vi "Curtin1_ViewType.vi"(10 "Settings":T2 {"mag/phase" items=["FRF", "rad phase unwrapped", "deg phase unwrapped", "rad phase wrapped", "deg phase wrapped", "White Plots", "MJ Map", "Real and Imaginary"]; "Bands" items=["No Bands", "", "Test2", "test3", "Test"]; "Smoothing" items=["No smoothing"=0, "1/4 semitone"=25, "1/2 semitone"=50, "1 semitone"=100, "2 semitones"=200, "Woodhouse"=19]; "View Type" items=["As measured", "Normalize", "Separate", "Complex Average", "Real Average", "Standard Deviation"]}, 11 "FRF in":cluster{dbl, "df":dbl, cdb[]}[](array[cluster])) -> (0 "Complex Out":cluster{dbl, "df":dbl, cdb[]}[](array[cluster]), 3 "FRF Out":cluster{"x0":dbl, "df":dbl, dbl[]}[](graph))   [LabVIEW 2022 SP3]
uses:
  GraphType.ctl
  Mic/Mic_Global.vi
  <vilib>/Analysis/NI_AALBase.lvlib
panel:
  out "Waveform Graph":cluster{dbl, "df":dbl, dbl[]}[](graph)
  out "Array":dbl[](array[numeric])
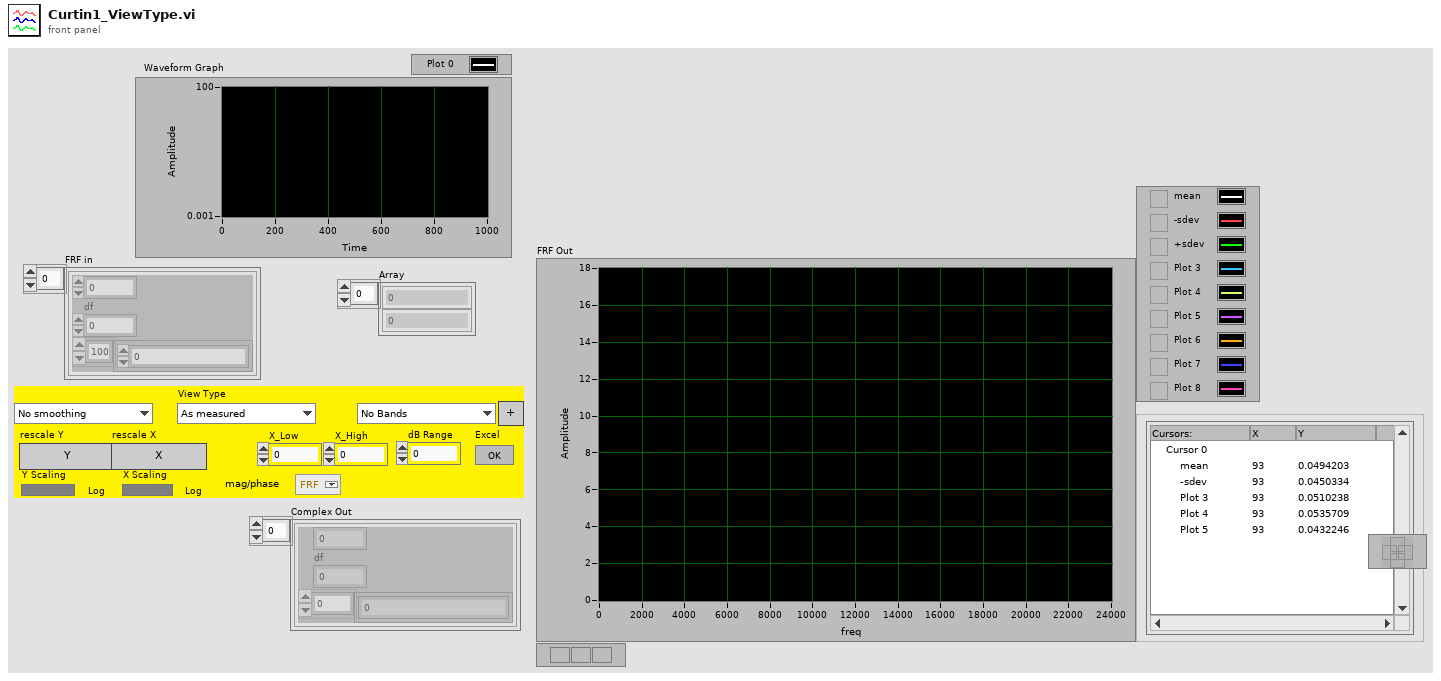
[diagram p1: front panel]
types:
  T1 = typedef "GraphType.ctl" = u16
  T2 = cluster{"View Type":u16, "Smoothing":u16, "Bands":u16, "New Band":bool, "rescale Y":bool, "rescale X":bool, "X_Low":dbl, "X_High":dbl, "dB Range":dbl, "Excel":bool, "Y Scaling":bool, "X Scaling":bool, "mag/phase":T1}
  T3 = cluster{"Alerts":bool, "Log X Axis":bool, "dB scale":bool, "Averaging":bool, "Fade":dbl, "Centroids?":bool, "line thickness":u8}
  T4 = typedef "PreferencesControl.ctl" = cluster{"Name of test":string, "Date":timestamp, "Location":string, "Template":string, "Soundcard":string, "resolution":u16, "Sampling rate":u16, "Ch1 Gain ":dbl, "Ch2 Gain":dbl, "Sample time (s)":dbl, "Pre-trigger (s)":dbl, "Hammer Threshold":dbl, "Positions":i16, "Taps/Position":i16, "Set Names":string, "Freq resolution":dbl, "Hammer cutoff":dbl, "Mic cutoff":dbl, "Double bounce ":dbl, "Hammer Cal":dbl, "dB Offset":dbl, "Accel Cal":dbl, "Vibrometer Cal":dbl, "Mic Cal":dbl, "Output":u16, "Voltage Cal":dbl, "Vibrometer Port":refnum<visa-resource-name>, "Range":u16, "High Pass":u16, "Bandwidth":u16, "X Range":cluster{"Minimum":dbl, "Maximum":dbl, "Increment":dbl, "Minor Increment":dbl, "Start":dbl}[], "Y Range":cluster{"Minimum":dbl, "Maximum":dbl, "Increment":dbl, "Minor Increment":dbl, "Start":dbl}[], "dB Spread":dbl, "Trigger":u16, "Ch_1":u8, "Ch_2":u8, "flip?":bool, "60Hz":bool, "Time offset":dbl, "Piezo Cal":dbl, "Default Notes":string}
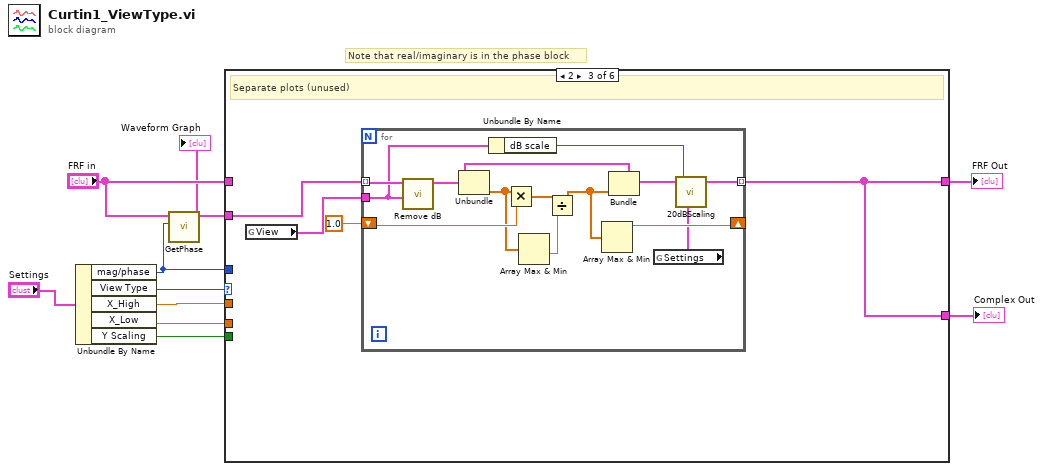
[diagram p0: block diagram]
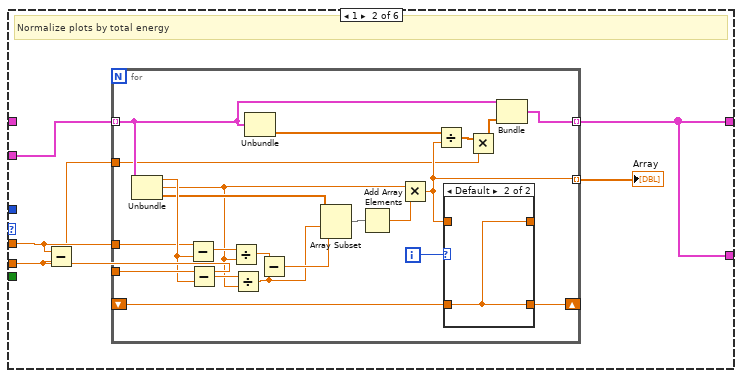
[diagram p3: hidden frame]
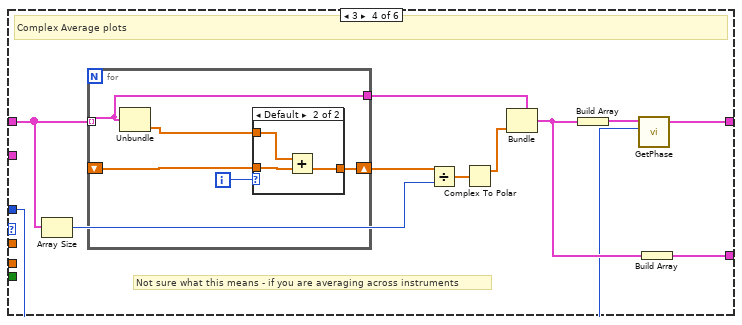
[diagram p5: hidden frame]
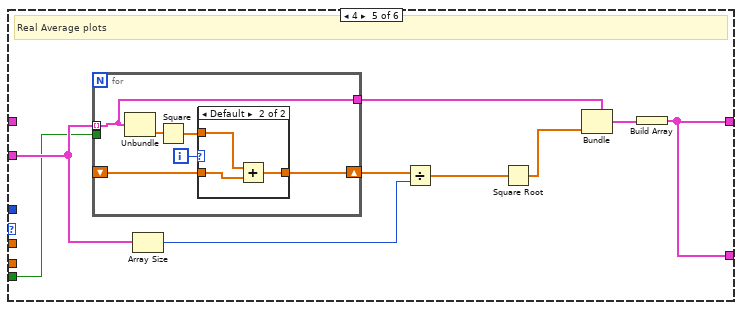
[diagram p7: hidden frame]
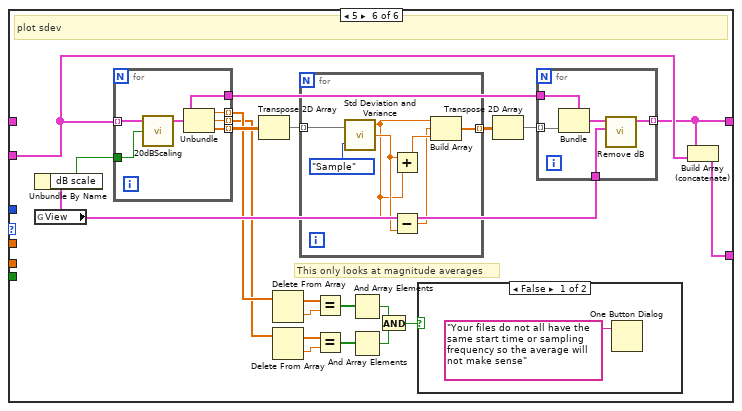
[diagram p9: hidden frame]
diagram:
  # "Note that real/imaginary is in the phase block"
  n1 = Unbundle By Name("Settings") -> ("mag/phase"=w4:T1, "View Type"=w9:u16, "X_High"=w7:dbl, "X_Low"=w8:dbl, "Y Scaling"=w3:bool)
  n2 = call "GetPhase.vi"("mag/phase"=w4, "FRF in"="FRF in") -> ("Array"=w1:cluster{dbl, "df":dbl, dbl[]}[])  [unwired: 9 in]
  "Waveform Graph" <- w1
  n3 = case shown="2" w9 {
    tunnel: "FRF in" -> [w12 _ _ w68 _ _]
    tunnel: [w11 w17 w44 w63 w82 w99] -> w2
    tunnel: w7 -> [_ w16 _ _ _ _]
    tunnel: w8 -> [_ w15 _ _ _ _]
    tunnel: [w12 w17 w44 w66 w82 w100] -> w6
    tunnel: w1 -> [w11 w13 w43 _ w81 w101]
    tunnel: w4 -> [_ _ _ w62 _ _]
    tunnel: w3 -> [_ _ _ _ w80 _]
    frame 0, Default {
    }
    frame 1 {
      # "Normalize plots by total energy"
      n4 = Subtract(x=w16, y=w15) -> (x-y=w14:dbl)
      n5 = for {
        tunnel: w13 -> [w20] mode=indexing
        tunnel: [w40] -> w17 mode=indexing
        tunnel: w15 -> [w28]
        tunnel: w16 -> [w27]
        shift-right: [w25] -> _
        shift-left: _ -> [w24]
        tunnel: [w21] -> w18 mode=indexing
        tunnel: w14 -> [w19]
        i -> [w26]
        n6 = Unbundle(w20) -> (w35:dbl, "df"=w23:dbl, w30:dbl[])
        n7 = Subtract(x=w27, y=w35) -> (x-y=w34:dbl)
        n8 = Subtract(x=w28, y=w35) -> (x-y=w36:dbl)
        n9 = Divide(x=w34, y=w23) -> (x/y=w29:dbl)
        n10 = Divide(x=w36, y=w23) -> (x/y=w31:dbl)
        n11 = Unbundle(w20) -> (w39:dbl[])  [unwired: 2 out]
        n12 = Subtract(x=w29, y=w31) -> (x-y=w32:dbl)
        n13 = Array Subset(array=w30, index=w31, length=w32) -> (w33:dbl[])
        n14 = Add Array Elements(numeric array=w33) -> (sum=w22:dbl)
        n15 = Multiply(x=w23, y=w22) -> (x*y=w21:dbl)
        n16 = Divide(x=w39, y=w21) -> (x/y=w38:dbl[])
        n17 = case shown="Default" w26 {
          tunnel: [w41 w42] -> _
          tunnel: w21 -> [w41 _]
          tunnel: [w41 w42] -> w25
          tunnel: w24 -> [_ w42]
          frame 0 {
          }
          frame Default {
          }
        }
        n18 = Multiply(x=w38, y=w19) -> (x*y=w37:dbl[])
        n19 = Bundle(cluster=w20, w37) -> (w40:cluster{dbl, "df":dbl, dbl[]})  [unwired: 2 in]
      }
      "Array" <- w18
    }
    frame 2 {
      # "Separate plots (unused)"
      n20 = global read "Mic_Global.vi" "View"() -> (w45:T3)
      n21 = for {
        tunnel: w43 -> [w56] mode=indexing
        shift-right: [w57] -> _
        shift-left: 1.0 -> [w59]
        tunnel: [w53] -> w44 mode=indexing
        tunnel: w45 -> [w52]
        n22 = call "Remove dB.vi"("View"=w52, "Average FRF in"=w56) -> ("Average FRF out"=w55:cluster{"x0":dbl, "df":dbl, dbl[]})  [unwired: 9 in]
        n23 = Unbundle(w55) -> (w49:dbl[])  [unwired: 2 out]
        n24 = Unbundle By Name(w52) -> ("dB scale"=w51:bool)
        n25 = Multiply(x=w49, y=w59) -> (x*y=w58:dbl[])
        n26 = Array Max & Min(array=w49) -> (min value=w50:dbl)  [unwired: 3 out]
        n27 = Divide(x=w58, y=w50) -> (x/y=w48:dbl[])
        n28 = Array Max & Min(array=w48) -> (max value=w57:dbl)  [unwired: 3 out]
        n29 = Bundle(cluster=w55, w48) -> (w54:cluster{"x0":dbl, "df":dbl, dbl[]})  [unwired: 2 in]
        n30 = global read "Mic_Global.vi" "Settings"() -> (w47:T4)
        n31 = call "20dBScaling.vi"("Average FRF in"=w54, "dB?"=w51, "Settings"=w47) -> ("Average FRF out"=w53:cluster{"x0":dbl, "df":dbl, dbl[]})  [unwired: 3 in, 1 out]
      }
    }
    frame 3 {
      # "Not sure what this means - if you are averaging across instruments"
      # "Complex Average plots"
      n32 = Array Size(array=w68) -> (size(s)=w67:i32)
      n33 = for {
        tunnel: w68 -> [w75] mode=indexing
        tunnel: [w75] -> w70
        shift-right: [w73] -> w69
        shift-left: _ -> [w72]
        i -> [w74]
        n34 = Unbundle(w75) -> (w71:cdb[])  [unwired: 2 out]
        n35 = case shown="Default" w74 {
          tunnel: [w76 w77] -> w73
          tunnel: w71 -> [w76 w78]
          tunnel: w72 -> [_ w79]
          frame 0 {
          }
          frame Default {
            n36 = Add(x=w78, y=w79) -> (x+y=w77:cdb[])
          }
        }
      }
      n37 = Divide(x=w69, y=w67) -> (x/y=w61:cdb[])
      n38 = Complex To Polar(r * e^(i*theta)=w61) -> (r=w60:dbl[])  [unwired: 1 out]
      n39 = Bundle(cluster=w70, w60) -> (w65:cluster{dbl, "df":dbl, cdb[]})  [unwired: 2 in]
      n40 = Build Array(w65) -> (w64:cluster{dbl, "df":dbl, cdb[]}[])
      n41 = call "GetPhase.vi"("mag/phase"=w62, "FRF in"=w64) -> ("Array"=w63:cluster{dbl, "df":dbl, dbl[]}[])  [unwired: 9 in]
      n42 = Build Array(w65) -> (w66:cluster{dbl, "df":dbl, cdb[]}[])
    }
    frame 4 {
      # "Real Average plots"
      n43 = for {
        tunnel: w81 -> [w89] mode=indexing
        tunnel: [w89] -> w88
        shift-right: [w93] -> w87
        shift-left: _ -> [w91]
        tunnel: w80 -> [_]
        i -> [w94]
        n44 = Unbundle(w89) -> (w92:dbl[])  [unwired: 2 out]
        n45 = Square(x=w92) -> (x^2=w90:dbl[])
        n46 = case shown="Default" w94 {
          tunnel: [w95 w96] -> w93
          tunnel: w90 -> [w95 w97]
          tunnel: w91 -> [_ w98]
          frame 0 {
          }
          frame Default {
            n47 = Add(x=w97, y=w98) -> (x+y=w96:dbl[])
          }
        }
      }
      n48 = Array Size(array=w81) -> (size(s)=w86:i32)
      n49 = Divide(x=w87, y=w86) -> (x/y=w85:dbl[])
      n50 = Square Root(x=w85) -> (sqrt(x)=w83:dbl[])
      n51 = Bundle(cluster=w88, w83) -> (w84:cluster{dbl, "df":dbl, dbl[]})  [unwired: 2 in]
      n52 = Build Array(w84) -> (w82:cluster{dbl, "df":dbl, dbl[]}[])
    }
    frame 5 {
      # "This only looks at magnitude averages"
      # "plot sdev"
      n53 = global read "Mic_Global.vi" "View"() -> (w115:T3)
      n54 = Unbundle By Name(w115) -> ("dB scale"=w116:bool)
      n55 = for {
        tunnel: w101 -> [w134] mode=indexing
        tunnel: [w133] -> w119
        tunnel: [w138] -> w118 mode=indexing
        tunnel: w116 -> [w137]
        tunnel: [w136] -> w112 mode=indexing
        tunnel: [w135] -> w105 mode=indexing
        n56 = call "20dBScaling.vi"("Average FRF in"=w134, "dB?"=w137) -> ("Average FRF out"=w133:cluster{"x0":dbl, "df":dbl, dbl[]})  [unwired: 4 in, 1 out]
        n57 = Unbundle(w133) -> ("x0"=w136:dbl, "df"=w135:dbl, w138:dbl[])
      }
      n58 = Transpose 2D Array(2D array=w118) -> (transposed array=w114:dbl[][])
      n59 = Delete From Array(array=w112) -> (deleted portion=w111:dbl, array with subset deleted=w110:dbl[])  [unwired: 2 in]
      n60 = Delete From Array(array=w105) -> (deleted portion=w106:dbl, array with subset deleted=w107:dbl[])  [unwired: 2 in]
      n61 = for {
        tunnel: w114 -> [w132] mode=indexing
        tunnel: [w128] -> w113 mode=indexing
        n62 = call <vilib>:"Std Deviation and Variance.vi"("X"=w132, "Weighting (Sample)"=enum16{"Sample", "Population"}."Sample") -> ("mean"=w129:dbl, "standard deviation"=w131:dbl)  [unwired: 1 out]
        n63 = Add(x=w131, y=w129) -> (x+y=w127:dbl)
        n64 = Subtract(x=w129, y=w131) -> (x-y=w126:dbl)
        n65 = Build Array(w129, w126, w127) -> (w128:dbl[])
      }
      n66 = Equal?(x=w110, y=w111) -> (x = y?=w109:bool[])
      n67 = Equal?(x=w107, y=w106) -> (x = y?=w108:bool[])
      n68 = And Array Elements(Boolean array=w109) -> (logical AND=w104:bool)
      n69 = And Array Elements(Boolean array=w108) -> (logical AND=w103:bool)
      n70 = And(x=w104, y=w103) -> (x .and. y?=w102:bool)
      n71 = case shown="False" w102 {
        frame False {
          n72 = One Button Dialog(message="Your files do not all have the same start time or sampling frequency so the average will not make sense") -> ()  [unwired: 1 in, 1 out]
        }
        frame True {
        }
      }
      n73 = Transpose 2D Array(2D array=w113) -> (transposed array=w117:dbl[][])
      n74 = for {
        tunnel: w119 -> [w125]
        tunnel: [w121] -> w99 mode=indexing
        tunnel: w117 -> [w124] mode=indexing
        tunnel: w115 -> [w123]
        n75 = Bundle(cluster=w125, w124) -> (w122:cluster{"x0":dbl, "df":dbl, dbl[]})  [unwired: 2 in]
        n76 = call "Remove dB.vi"("View"=w123, "Average FRF in"=w122) -> ("Average FRF out"=w121:cluster{"x0":dbl, "df":dbl, dbl[]})  [unwired: 9 in]
      }
      n77 = Build Array (concatenate)(w99, w101) -> (w100:cluster{"x0":dbl, "df":dbl, dbl[]}[])
    }
  }
  "Complex Out" <- w6
  "FRF Out" <- w2
